vi "Enable Source Output.vi"(8 "error in (no error)":errorcluster, 9 "Output Mode (0: Turn off)":i32(ring) items=["Turn off", "Turn On", "High-Z"], 10 "Source Measure Unit Channel (0: Channel A)":i32(ring) items=["Channel A", "Channel B"], 11 "VISA resource name":refnum<visa-resource-name>) -> (0 "error out":errorcluster, 3 "VISA resource name out":refnum<visa-resource-name>)   [LabVIEW 2017, in "Keithley 2600 Series.lvlib"]
doc: "Enables or disables the source output."
uses:
  <instrlib>/Keithley 2600 Series/Keithley 2600 Series.lvlib
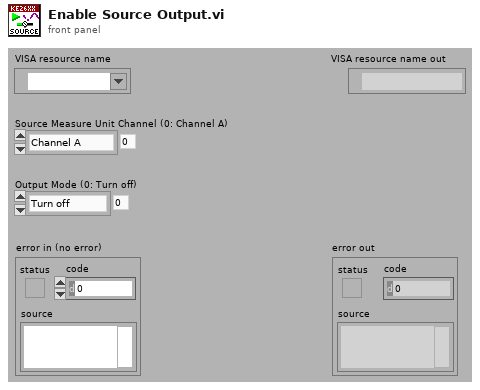
[diagram p1: front panel]
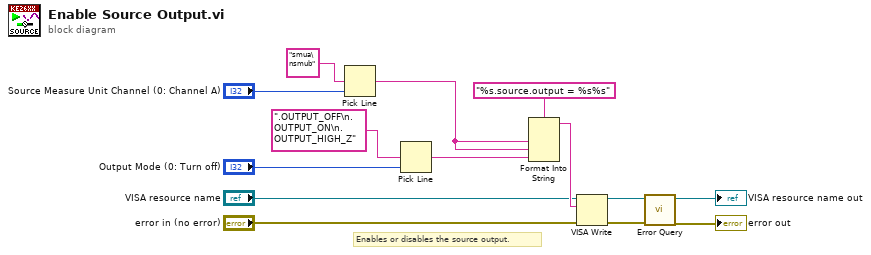
[diagram p0: block diagram]
diagram:
  # "Enables or disables the source output."
  n1 = Pick Line(multi-line string="smua\nsmub", line index="Source Measure Unit Channel (0: Channel A)") -> (output string=w4:string)  [unwired: 1 in]
  n2 = Pick Line(multi-line string=".OUTPUT_OFF\n.OUTPUT_ON\n.OUTPUT_HIGH_Z", line index="Output Mode (0: Turn off)") -> (output string=w3:string)  [unwired: 1 in]
  n3 = Format Into String(format string="%s.source.output = %s%s", w4, w4, w3) -> (resulting string=w13:string)  [unwired: 2 in, 1 out]
  n4 = VISA Write(VISA resource name="VISA resource name", write buffer=w13, error in (no error)="error in (no error)") -> (VISA resource name out=w10:refnum<visa-resource-name>, error out=w9:errorcluster)  [unwired: 1 out]
  n5 = call <instrlib>:"Error Query.vi"("error in (no error)"=w9, "VISA resource name"=w10) -> ("error out"=→"error out":errorcluster, "VISA resource name out"=→"VISA resource name out":refnum<visa-resource-name>)  [unwired: 6 in, 2 out]
